vi "calc_BOC_ampl_koef.vi"(8 "error_in":errorcluster, 9 "boc_data":sgl[](array[numeric]), 10 "meas":dbl[](array[numeric])) -> (0 "error_out":errorcluster, 3 "koef":dbl[](array[numeric]))   [LabVIEW 2017]
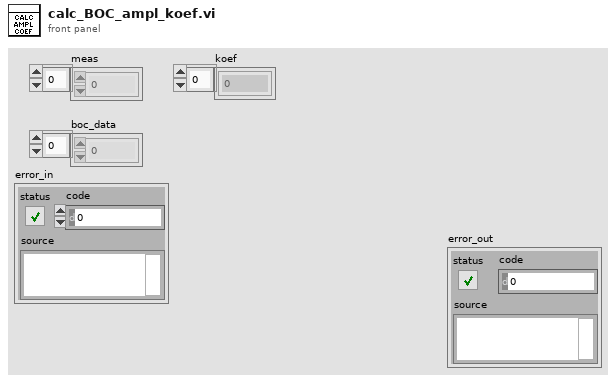
[diagram p1: front panel]
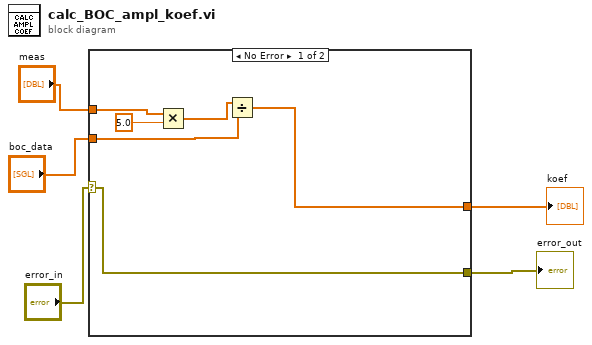
[diagram p0: block diagram]
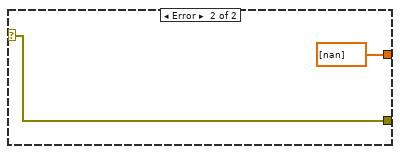
[diagram p2: hidden frame]
diagram:
  n1 = case shown="No Error" "error_in" {
    selector: "error_in" -> [w6 w13]
    tunnel: [w11 dbl[] [nan]] -> w5
    tunnel: "boc_data" -> [w10 _]
    tunnel: "meas" -> [w7 _]
    tunnel: [w6 w13] -> w2
    frame No Error {
      n2 = Multiply(x=w7, y=5.0) -> (x*y=w9:dbl[])
      n3 = Divide(x=w9, y=w10) -> (x/y=w11:dbl[])
    }
    frame Error {
    }
  }
  "koef" <- w5
  "error_out" <- w2
